vi "Icon Test VI.vi"() -> ()   [LabVIEW 2013]
uses:
  <vilib>/LabVIEW Icon API/lv_icon/Controls/BodyText.ctl
  <vilib>/LabVIEW Icon API/lv_icon/Controls/Font.ctl
  <vilib>/LabVIEW Icon API/lv_icon/Controls/Alignment.ctl
panel:
  out "VI Path":path
  out "Body Text":T1 {"Body Text Spec"."Alignment" items=["left", "center", "right"]}
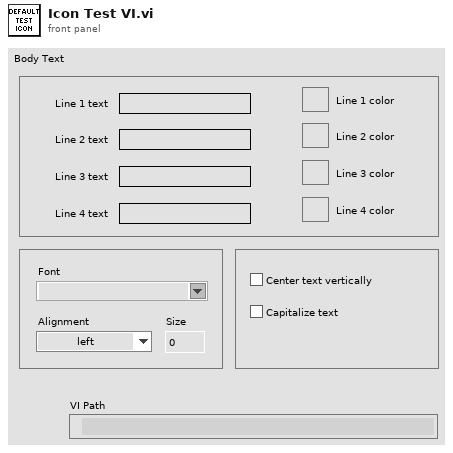
[diagram p1: front panel]
types:
  T1 = typedef "BodyText.ctl" = cluster{"Line 1 text":string, "Line 2 text":string, "Line 3 text":string, "Line 4 text":string, "Line 1 color":u32, "Line 2 color":u32, "Line 3 color":u32, "Line 4 color":u32, "Body Text Spec":cluster{"Font":T2, "Alignment":T3, "Size":u8}, "Center text vertically":bool, "Capitalize Text":bool}
  T2 = typedef "Font.ctl" = string
  T3 = typedef "Alignment.ctl" = u16
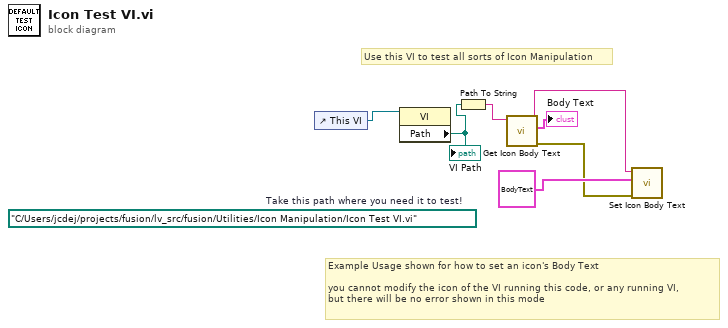
[diagram p0: block diagram]
diagram:
  (unwired) path "C:/Users/jcdej/projects/fusion/lv_src/fusion/Utilities/Icon Manipulation/Icon Test VI.vi"  # Take this path where you need it to test!
  # "Example Usage shown for how to set an icon's Body Text\n\nyou cannot modify the icon of the VI running this code, or any running VI,\nbut there will be no error shown in this mode"
  # "Use this VI to test all sorts of Icon Manipulation"
  n1 = control-ref of="This VI"() -> (w7:refnum<vi>)
  n2 = property class="VI"(reference=w7) -> ("Path"=w2:path)  [unwired: 1 in, 2 out]
  "VI Path" <- w2
  n3 = Path To String(path=w2) -> (string=w1:string)
  n4 = call "Get Icon Body Text.vi"("VI Path"=w1) -> ("error out"=w3:errorcluster, "Body Text"=→"Body Text":T1, "VI Path (dup)"=w4:string)  [unwired: 8 in]
  n5 = call "Set Icon Body Text.vi"("error in (no error)"=w3, "Body Text"=T1 {"Line 1 text"="default", "Line 2 text"="test", "Line 3 text"="icon", "Line 4 text"="", "Line 1 color"=0, "Line 2 color"=0, "Line 3 color"=0, "Line 4 color"=0, "Body Text Spec"={"Font"="Small Fonts", "Alignment"=1, "Size"=9}, "Center text vertically"=TRUE, "Capitalize Text"=TRUE}, "VI Path"=w4) -> ()  [unwired: 8 in, 1 out]
